vi "terminate.vi"(8 "error in (no error)":errorcluster, 11 "DL090211FrameImageAssembler in":refnum<class "ImageAssemblerDL090211Frame.lvclass">) -> (0 "error out":errorcluster, 3 "DL090211FrameImageAssembler out":refnum<class "ImageAssemblerDL090211Frame.lvclass">)   [LabVIEW 2010, in "ImageAssemblerDL090211Frame.lvclass"]
uses:
  ImageAssemblerDL090211Frame.lvclass
  common/arrays/pixel_raw_data_array.ctl
  ImageAssemblerDL090211Frame.lvclass/ImageAssemblerDL090211Frame.ctl
  common/classes/Image/Image/Image.lvclass
  ImageAssemblerDL090211Scaffold/ImageAssemblerDL090211Scaffold/ImageAssemblerDL090211Scaffold.lvclass
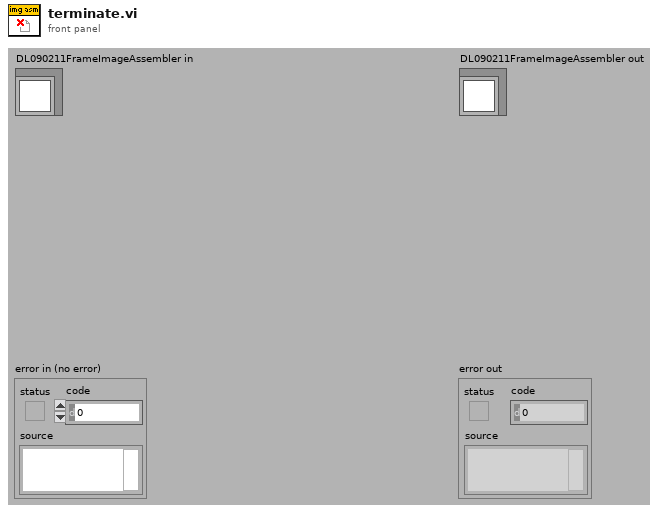
[diagram p1: front panel]
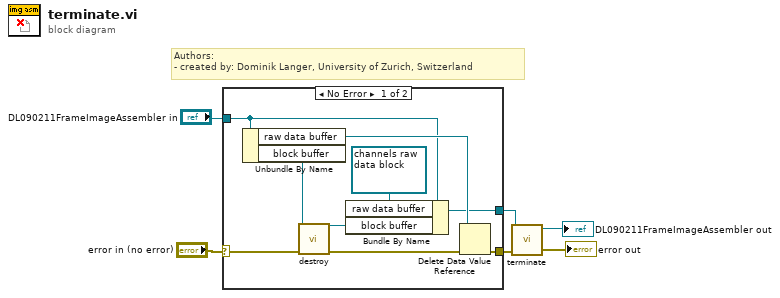
[diagram p0: block diagram]
diagram:
  # "Authors: \n- created by: Dominik Langer, University of Zurich, Switzerland"
  n1 = case shown="No Error" "error in (no error)" {
    selector: "error in (no error)" -> [w7 w17]
    tunnel: [w11 w17] -> w2
    tunnel: [w9 w16] -> w4
    tunnel: "DL090211FrameImageAssembler in" -> [w10 w16]
    frame No Error {
      n2 = Unbundle By Name(w10) -> ("raw data buffer"=w13:refnum<data-value>, "block buffer"=w15:refnum<class "Image.lvclass">)
      n3 = call-dynamic "destroy.vi"("error in (no error)"=w7, "Image in"=w15) -> ("error out"=w12:errorcluster, "Image out"=w14:refnum<class "Image.lvclass">)  [unwired: 8 out]
      n4 = Bundle By Name(cluster=w10, "raw data buffer"=refnum<data-value> refnum ("data value reference"), "block buffer"=w14) -> (w9:refnum<class "ImageAssemblerDL090211Frame.lvclass">)
      n5 = Delete Data Value Reference(data value reference=w13, error in=w12) -> (error out=w11:errorcluster)  [unwired: 1 out]
    }
    frame Error {
    }
  }
  n6 = call-parent "terminate.vi"("error in (no error)"=w2, "DL090211ImageAssemblerScaffold in"=w4) -> ("error out"=→"error out":errorcluster, "DL090211ImageAssemblerScaffold out"=→"DL090211FrameImageAssembler out":refnum<class "ImageAssemblerDL090211Frame.lvclass">)  [unwired: 8 out]
